vi "svetofor.vi"() -> ()   [LabVIEW 2017]
uses:
  <vilib>/userdefined/High Color/IMAQdx.ctl
  <vilib>/vision/driver/NI_Vision_Acquisition_Software.lvlib
panel:
  out "error out":errorcluster
  in  "error in":errorcluster
  out "Image":T1(plugin-control)
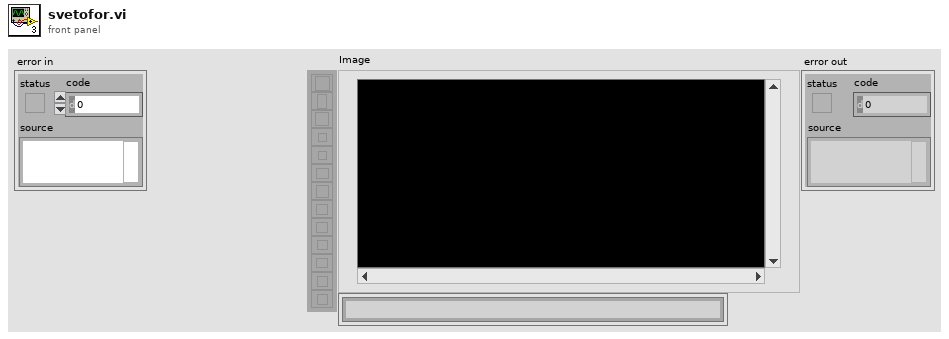
[diagram p1: front panel]
types:
  T1 = typedef "IMAQ Image.ctl" = refnum<image>
  T2 = typedef "IMAQdx.ctl" = refnum<k21>
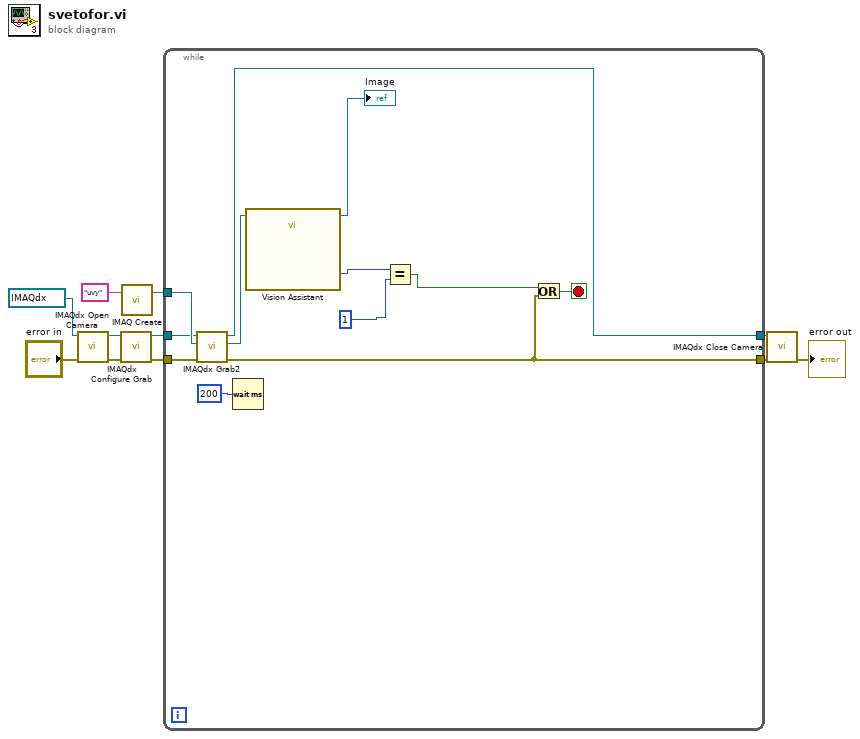
[diagram p0: block diagram]
diagram:
  n1 = call <vilib>:"IMAQdx Open Camera.vi"("error in"="error in", "Session In"=T2 "cam0") -> ("error out"=w8:errorcluster, "Session Out"=w5:T2)  [unwired: 8 in]
  n2 = call <vilib>:"IMAQdx Configure Grab.vi"("error in"=w8, "Session In"=w5) -> ("error out"=w7:errorcluster, "Session Out"=w4:T2)  [unwired: 8 in]
  n3 = call "IMAQ Create"("Image Name"="uvy") -> ("New Image"=w6:T1)  [unwired: 4 in, 1 out]
  n4 = while {
    tunnel: w7 -> [w23]
    tunnel: w6 -> [w22]
    tunnel: w4 -> [w21]
    tunnel: [w20] -> w3
    tunnel: [w16] -> w11
    stop <- w14 stop-if-true
    n5 = call <vilib>:"IMAQdx Grab2.vi"("error in"=w23, "Image In"=w22, "Session In"=w21) -> ("error out"=w16:errorcluster, "Image Out"=w19:T1, "Session Out"=w20:T2)  [unwired: 5 in, 1 out]
    n6 = Wait (ms)(milliseconds to wait=u32 200) -> ()  [unwired: 1 out]
    n7 = call "Vision Assistant"("Image In"=w19) -> ("Image Out"=→"Image":T1, "Number of Matches (Color Location 1)"=w12:i32)  [unwired: 24 in, 1 out]
    n8 = Equal?(x=w12, y=1 ("index")) -> (x = y?=w15:bool)
    n9 = Or(x=w15, y=w16) -> (x .or. y?=w14:bool)
  }
  n10 = call <vilib>:"IMAQdx Close Camera.vi"("error in"=w11, "Session In"=w3) -> ("error out"=→"error out":errorcluster)  [unwired: 9 in]
